vi "rs3 get api version.vi"(8 "error in (no error)":errorcluster) -> (0 "error out":errorcluster, 1 "error":u64, 3 "api_version":i32=20000)   [LabVIEW 2019, in "libRealSense3.lvlib"]
doc: "This has to be the first call to initiate libRealSense. \nThe input is the Version Check for the libRealSense, and the output is the Context that needs to be passed to Device Count and Get Device."
uses:
  libRealSense3.lvlib
  Intel RealSense SDK 2.0/bin/x86/realsense2.dll
panel:
  # "RS2 Get API Version"
  # "(C) Intel Corp.,  AGJ"
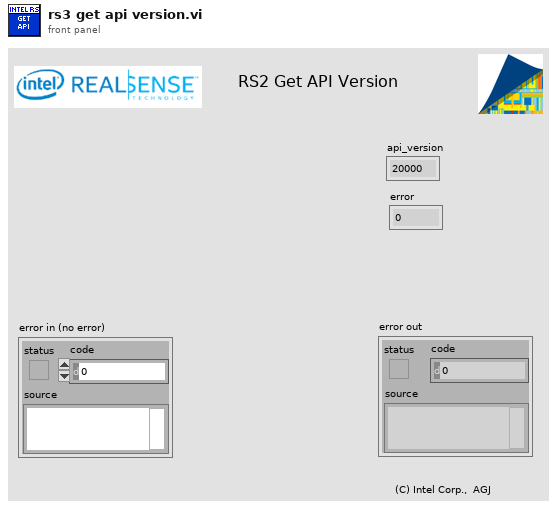
[diagram p1: front panel]
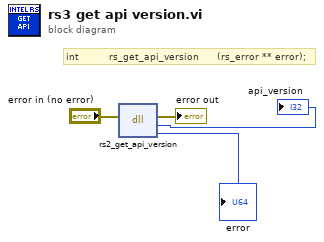
[diagram p0: block diagram]
diagram:
  # "int          rs_get_api_version      (rs_error ** error);"
  n1 = dll-call lib="C:/Program Files (x86)/Intel RealSense SDK 2.0/bin/x86/realsense2.dll" fn="rs2_get_api_version"(error in="error in (no error)") -> (error out=→"error out":errorcluster, "return type"=→"api_version":i32, "error"=→"error":u64)  [unwired: 3 in, 1 out]
